vi "do_output.vi"(6 "In clock":bool, 8 "In value":bool, 9 "Out active":bool, 10 "Out value":bool, 11 "Out pin":refnum<k21>) -> (1 "Stuck":bool)   [LabVIEW 2010]
panel:
  # "True if the line is stuck (has the wrong value.)"
  # "Output is represented by two signals \"Out active\", which indicates whether we should be in control of that bus line, and \"Out value\", which is the value it should have when active."
  # "\"In value\" is the value read from the bus, which should equal \"Out value\" at the specified \"In clock\" edge, if the line is active."
  # "Grouping of common processing for SDA and SCL outputs.  As well as doing the output itself, we also check for the line being stuck at the incorrect value, which would indicate bus contention or a fault."
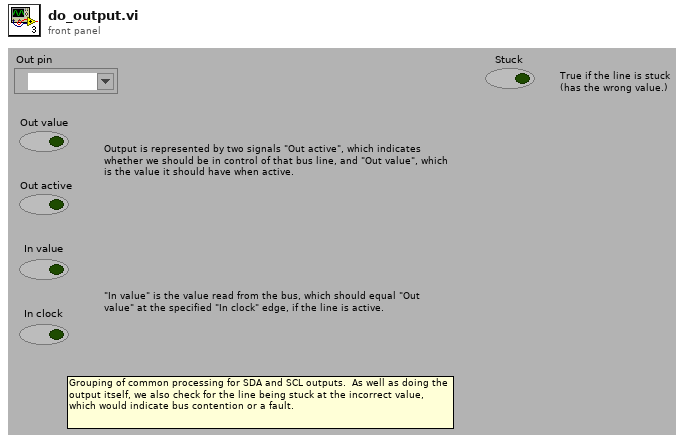
[diagram p1: front panel]
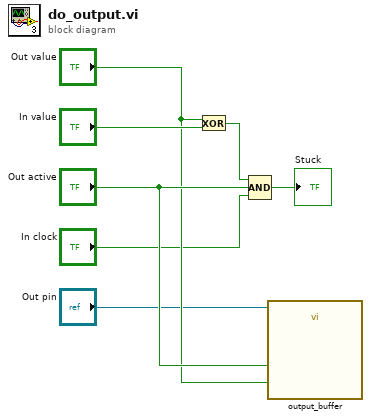
[diagram p0: block diagram]
diagram:
  n1 = Exclusive Or(1:"In value", 2:"Out value") -> (0:w5:bool)
  n2 = Compound Arithmetic op=AND(w5, "Out active", "In clock") -> (→"Stuck":bool)
  n3 = call "output_buffer.vi"("Line active"="Out active", "Line out"="Out value", "Out pin"="Out pin") -> ()
